vi "Close References.vi"(8 "error in":errorcluster, 11 "References":T1) -> (0 "error out":errorcluster)   [LabVIEW 2020]
uses:
  Controls/Car Wash References.ctl
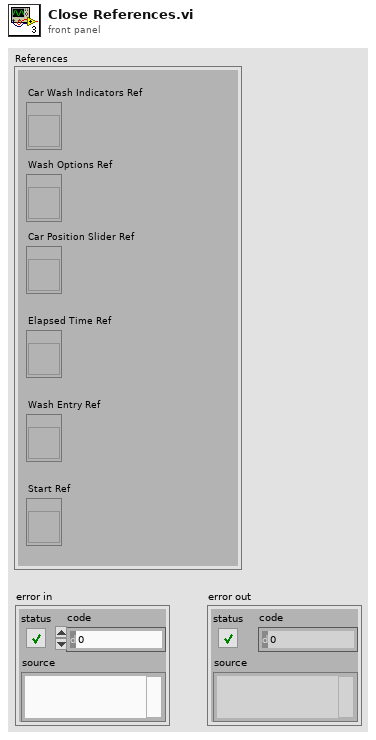
[diagram p1: front panel]
types:
  T1 = typedef "Car Wash References.ctl" = cluster{"Car Wash Indicators Ref":refnum<vi>, "Wash Options Ref":refnum<vi>, "Car Position Slider Ref":refnum<vi>, "Elapsed Time Ref":refnum<vi>, "Wash Entry Ref":refnum<vi>, "Start Ref":refnum<vi>}
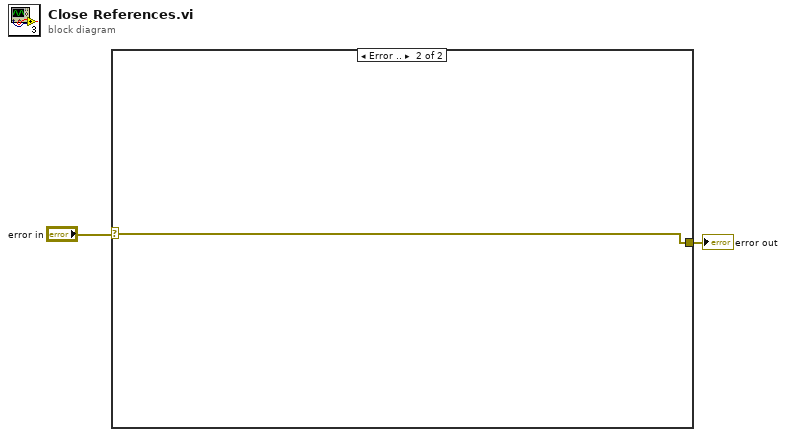
[diagram p0: block diagram]
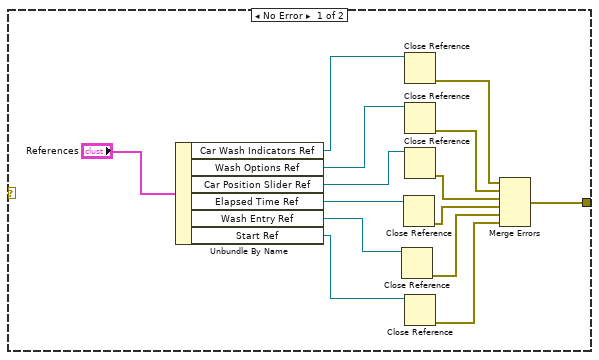
[diagram p2: hidden frame]
diagram:
  n1 = case shown="Error .." "error in" {
    selector: "error in" -> [_ w17]
    tunnel: [w3 w17] -> w2
    frame No Error {
      n2 = Unbundle By Name("References") -> ("Car Wash Indicators Ref"=w11:refnum<vi>, "Wash Options Ref"=w12:refnum<vi>, "Car Position Slider Ref"=w13:refnum<vi>, "Elapsed Time Ref"=w14:refnum<vi>, "Wash Entry Ref"=w15:refnum<vi>, "Start Ref"=w16:refnum<vi>)
      n3 = Close Reference(reference=w15) -> (error out=w5:errorcluster)  [unwired: 1 in]
      n4 = Close Reference(reference=w14) -> (error out=w6:errorcluster)  [unwired: 1 in]
      n5 = Close Reference(reference=w11) -> (error out=w9:errorcluster)  [unwired: 1 in]
      n6 = Close Reference(reference=w12) -> (error out=w8:errorcluster)  [unwired: 1 in]
      n7 = Close Reference(reference=w13) -> (error out=w7:errorcluster)  [unwired: 1 in]
      n8 = Close Reference(reference=w16) -> (error out=w4:errorcluster)  [unwired: 1 in]
      n9 = Merge Errors(w9, w8, w7, w6, w5, w4) -> (w3:errorcluster)
    }
    frame Error {
    }
  }
  "error out" <- w2
